vi "CreateGlobalEvents.vi"   [LabVIEW 2017]
uses:
  Globals/globals.vi
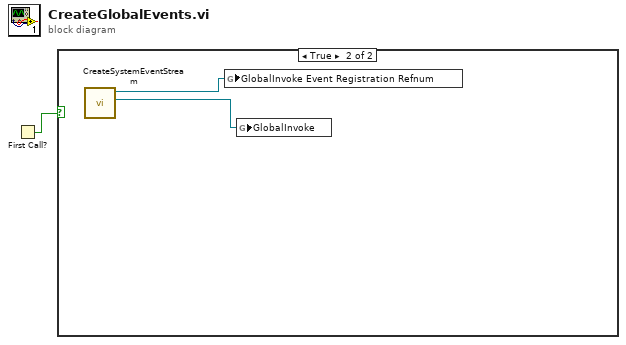
[diagram p0: block diagram]
diagram:
  n1 = First Call?() -> (First Call?: T/F=w1:bool)
  n2 = case shown="True" w1 {
    frame False {
    }
    frame True {
      n3 = call "CreateSystemEventStream.vi"() -> ("Event Stream Out"=w2:refnum<user-event>, "Event Registration Refnum out"=w3:refnum<event-registration>)  [unwired: 10 in]
      n4 = global write "globals.vi" "GlobalInvoke Event Registration Refnum"(w3) -> ()
      n5 = global write "globals.vi" "GlobalInvoke"(w2) -> ()
    }
  }
